vi "Client_next.vi"(10 "lambda":dbl=0.1 format="%#_13g", 11 "Time of previous":dbl) -> (3 "Client":T1)   [LabVIEW 2014, in "LukiBrary.lvlib"]
doc: "Otrzymuje czas poprzedniego klienta, parametr lambda (oczekiwaną liczbę klientów na jednostkę czasu [SEK]). Losuje (tworzy) klienta."
uses:
  LukiBrary.lvlib
  Client.ctl
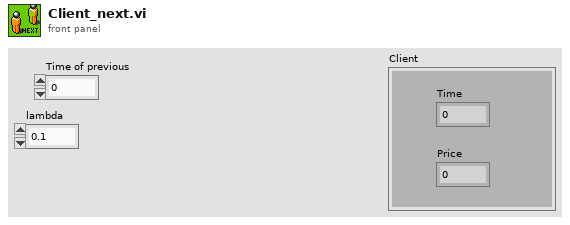
[diagram p1: front panel]
types:
  T1 = typedef "LukiBrary.lvlib/Client.ctl" = cluster{"Time":dbl, "Price":dbl}
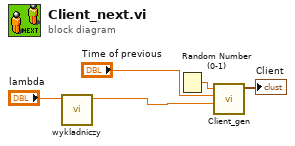
[diagram p0: block diagram]
diagram:
  n1 = call "wykladniczy.vi"("lambda"="lambda") -> ("X~wykładniczy"=w1:dbl)  [unwired: 10 in]
  n2 = Random Number (0-1)() -> (number: 0 to 1=w4:dbl)
  n3 = call "Client_gen.vi"("Różnica"=w1, "Time"="Time of previous", "Price"=w4) -> ("Client"=→"Client":T1)  [unwired: 8 in]
